vi "ConfigureChannelPhaseStatus.vi"(8 "shared data group exist?":bool, 9 "AssetNodes":T5[](array[typedef]), 10 "AllChannels":T3[](array[typedef]), 11 "ChannelModel":T3) -> (2 "valid":bool, 3 "DataGroup ChannelStatus Out":T1[](array[typedef]))   [LabVIEW 2017, in "McsaTestPanel.lvlib"]
uses:
  <vilib>/addons/InsightCM/Devices/Shared/Mcsa/McsaTestPanel/McsaTestPanel.lvlib
  <vilib>/addons/InsightCM/MessageBus/Base/controls/AssetNode.ctl
  <vilib>/addons/InsightCM/MessageBus/Base/controls/AssetState.ctl
  <vilib>/addons/InsightCM/MessageBus/Base/controls/KeyValuePair.ctl
  <vilib>/addons/InsightCM/MessageBus/Base/controls/OperatingState.ctl
  <vilib>/addons/InsightCM/MessageBus/Base/controls/Trigger.ctl
  <vilib>/addons/InsightCM/MessageBus/Base/controls/Condition.ctl
  <vilib>/addons/InsightCM/MessageBus/Base/controls/Metric.ctl
  <vilib>/addons/InsightCM/MessageBus/Base/controls/TrendAlarmRule.ctl
  <vilib>/addons/InsightCM/MessageBus/Base/controls/TrendAlarmLevel.ctl
  <vilib>/addons/InsightCM/MessageBus/Base/controls/AlarmAction.ctl
  <vilib>/addons/InsightCM/MessageBus/Base/controls/AssetNodeReference.ctl
  <vilib>/addons/InsightCM/MessageBus/Base/controls/R2_Channel.ctl
  <vilib>/addons/InsightCM/Devices/Shared/Mcsa/McsaTestPanel/controls/ChannelStatus.ctl
  <vilib>/addons/InsightCM/Utilities/PropertyHelpers/PropertyHelpers.lvlib
  <vilib>/addons/InsightCM/Utilities/DeviceModelHelpers/DeviceModelHelpers.lvlib
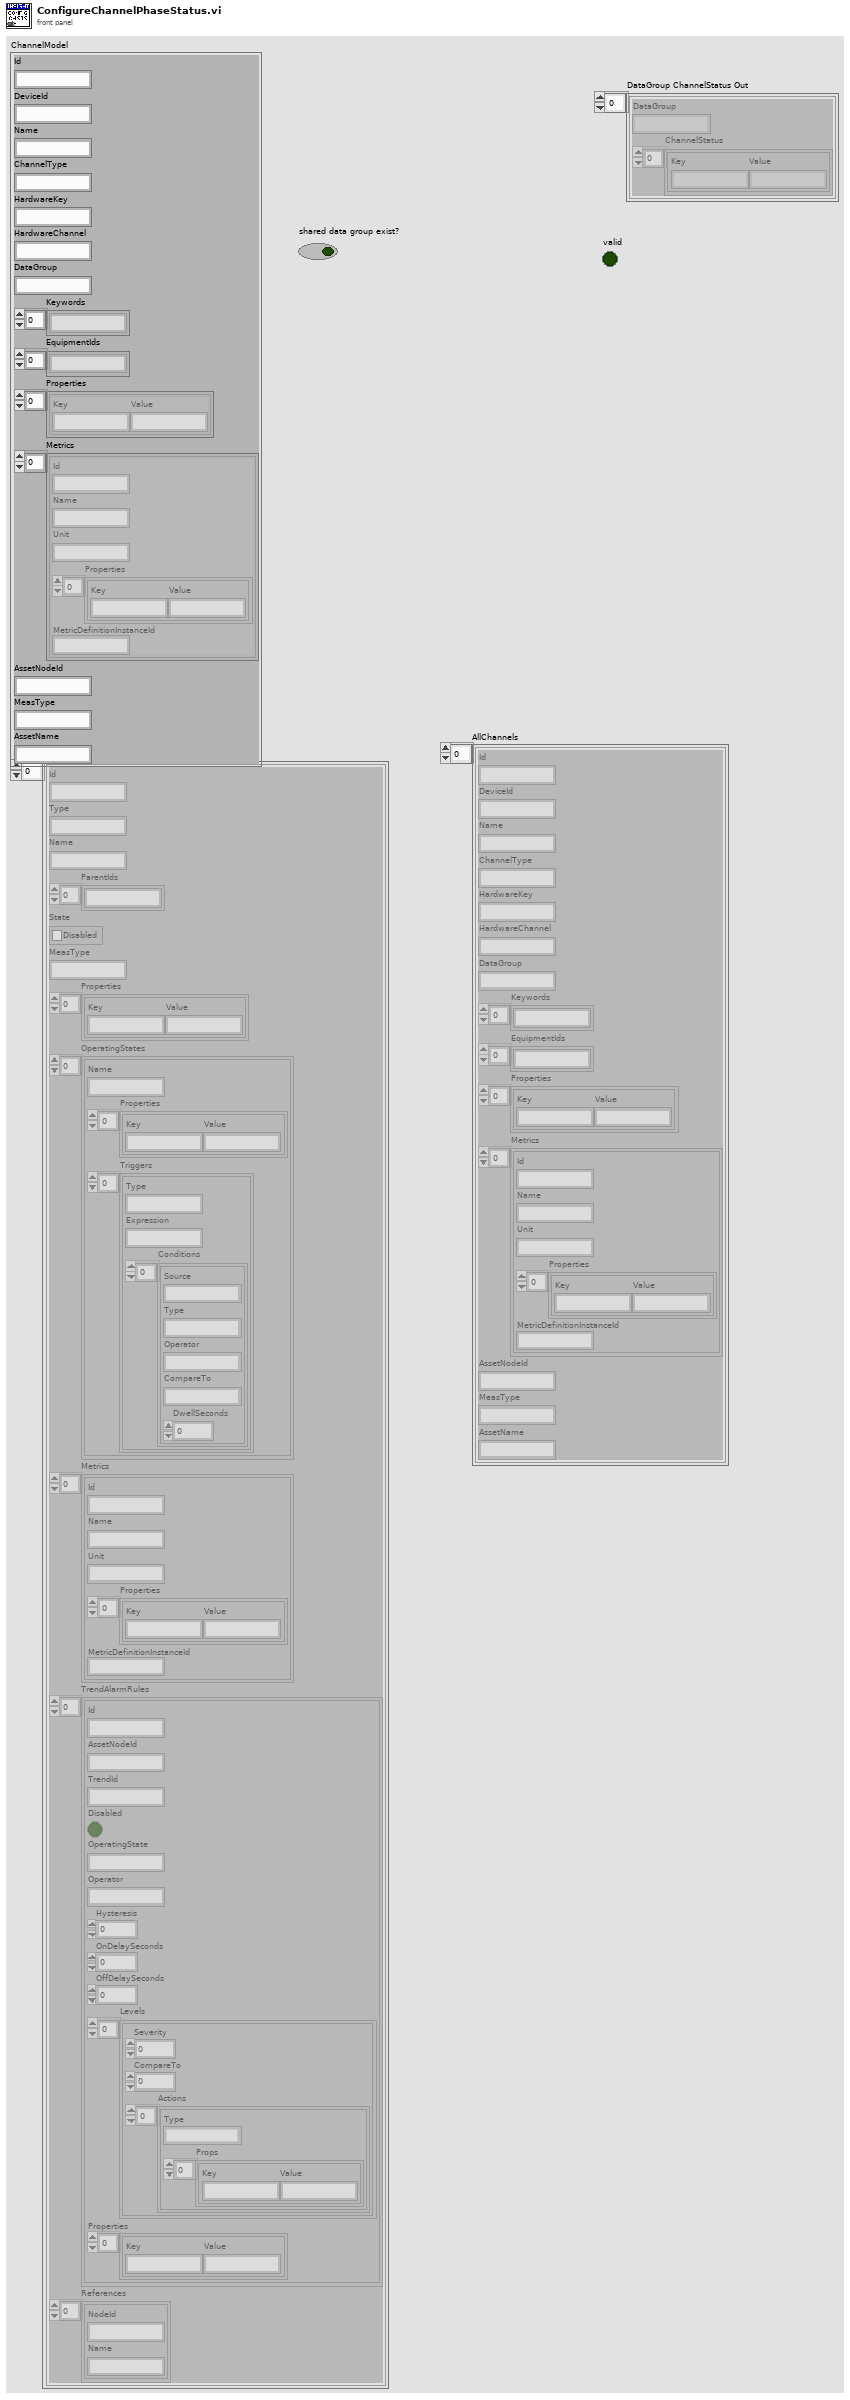
[diagram p1: front panel]
types:
  T1 = typedef "McsaTestPanel.lvlib/ChannelStatus.ctl" = cluster{"DataGroup":string, "ChannelStatus":T2[]}
  T2 = typedef "KeyValuePair.ctl" = cluster{"Key":string, "Value":string}
  T3 = typedef "R2_Channel.ctl" = cluster{"Id":string, "DeviceId":string, "Name":string, "ChannelType":string, "HardwareKey":string, "HardwareChannel":string, "DataGroup":string, "Keywords":string[], "EquipmentIds":string[], "Properties":T2[], "Metrics":T4[], "AssetNodeId":string, "MeasType":string, "AssetName":string}
  T4 = typedef "Metric.ctl" = cluster{"Id":string, "Name":string, "Unit":string, "Properties":T2[], "MetricDefinitionInstanceId":string}
  T5 = typedef "AssetNode.ctl" = cluster{"Id":string, "Type":string, "Name":string, "ParentIds":string[], "State":T6, "MeasType":string, "Properties":T2[], "OperatingStates":T7[], "Metrics":T4[], "TrendAlarmRules":T10[], "References":T13[]}
  T6 = typedef "AssetState.ctl" = cluster{"Disabled":bool}
  T7 = typedef "OperatingState.ctl" = cluster{"Name":string, "Properties":T2[], "Triggers":T8[]}
  T8 = typedef "Trigger.ctl" = cluster{"Type":string, "Expression":string, "Conditions":T9[]}
  T9 = typedef "Condition.ctl" = cluster{"Source":string, "Type":string, "Operator":string, "CompareTo":string, "DwellSeconds":dbl}
  T10 = typedef "TrendAlarmRule.ctl" = cluster{"Id":string, "AssetNodeId":string, "TrendId":string, "Disabled":bool, "OperatingState":string, "Operator":string, "Hysteresis":dbl, "OnDelaySeconds":dbl, "OffDelaySeconds":dbl, "Levels":T11[], "Properties":T2[]}
  T11 = typedef "TrendAlarmLevel.ctl" = cluster{"Severity":i32, "CompareTo":dbl, "Actions":T12[]}
  T12 = typedef "AlarmAction.ctl" = cluster{"Type":string, "Props":T2[]}
  T13 = typedef "AssetNodeReference.ctl" = cluster{"NodeId":string, "Name":string}
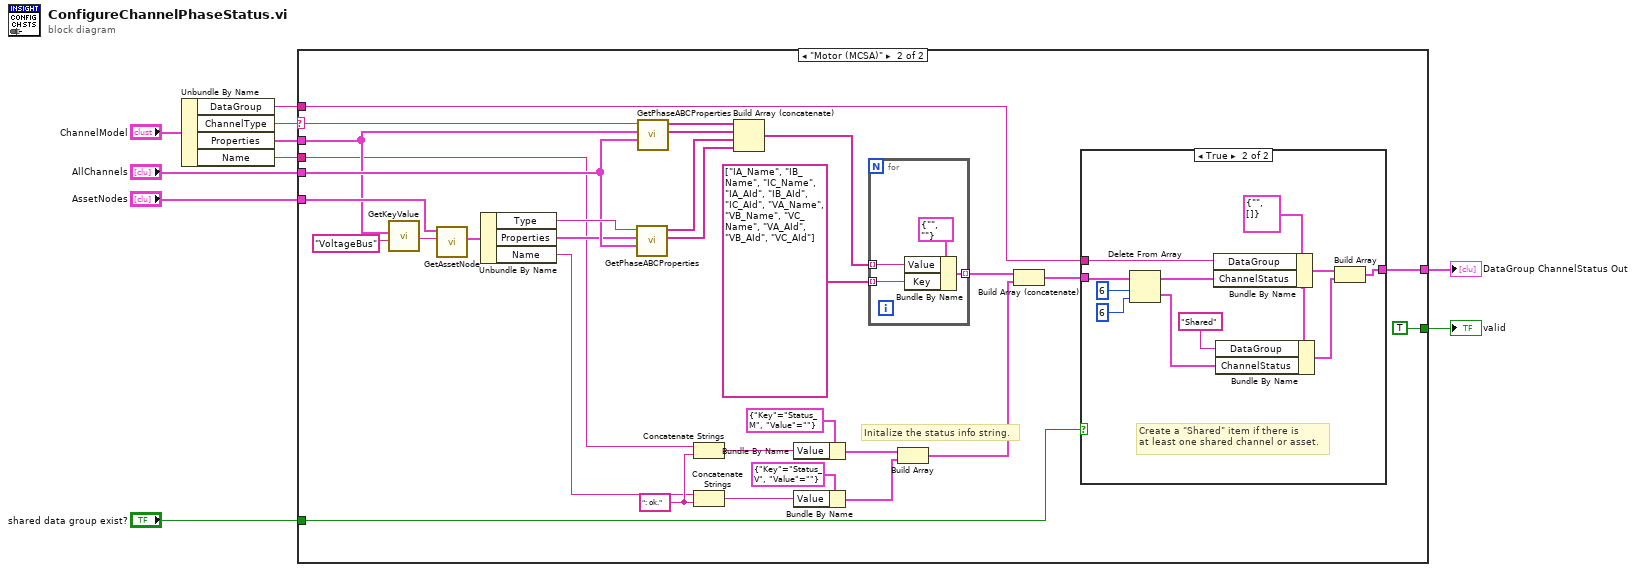
[diagram p0: block diagram]
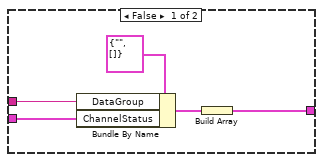
[diagram p3: hidden frame]
diagram:
  n1 = Unbundle By Name("ChannelModel") -> ("DataGroup"=w5:string, "ChannelType"=w6:string, "Properties"=w7:T2[], "Name"=w2:string)
  n2 = case shown="\"Motor (MCSA)\"" w6 {
    selector: w6 -> [_ w41]
    tunnel: w7 -> [_ w35]
    tunnel: "AllChannels" -> [_ w36]
    tunnel: "AssetNodes" -> [_ w39]
    tunnel: w5 -> [_ w13]
    tunnel: [_ w29] -> w3
    tunnel: "shared data group exist?" -> [_ w12]
    tunnel: w2 -> [_ w19]
    tunnel: [_ TRUE ("valid")] -> w1
    frame Default {
    }
    frame "Motor (MCSA)" {
      w20 = ": ok." ("string")
      # "Initalize the status info string."
      n3 = call <vilib>:"GetKeyValue.vi"("key"="VoltageBus", "key value pairs"=w35) -> ("value"=w23:string)  [unwired: 7 in, 2 out]
      n4 = call <vilib>:"GetAssetNode.vi"("node id"=w23, "nodes in"=w39) -> ("AssetNode"=w38:T5)  [unwired: 7 in, 2 out]
      n5 = Unbundle By Name(w38) -> ("Type"=w37:string, "Properties"=w34:T2[], "Name"=w18:string)
      n6 = call <vilib>:"GetPhaseABCProperties.vi"("Channels"=w36, "Channel Properties"=w34, "ChannelType"=w37) -> ("AssetIdABC"=w14:string[], "AssetNameABC"=w15:string[])  [unwired: 6 in, 1 out]
      n7 = call <vilib>:"GetPhaseABCProperties.vi"("Channels"=w36, "Channel Properties"=w35, "ChannelType"=w41) -> ("AssetIdABC"=w16:string[], "AssetNameABC"=w17:string[])  [unwired: 6 in, 1 out]
      n8 = Concatenate Strings(w19, w20) -> (w21:string)
      n9 = Concatenate Strings(w18, w20) -> (w22:string)
      n10 = Build Array (concatenate)(w17, w16, w15, w14) -> (w33:string[])
      n11 = Bundle By Name(cluster=T2 {"Key"="Status_M", "Value"=""}, "Value"=w21) -> (w26:T2)
      n12 = Bundle By Name(cluster=T2 {"Key"="Status_V", "Value"=""}, "Value"=w22) -> (w25:T2)
      n13 = for {
        tunnel: w33 -> [w60] mode=indexing
        tunnel: string[] ["IA_Name", "IB_Name", "IC_Name", "IA_AId", "IB_AId", "IC_AId", "VA_Name", "VB_Name", "VC_Name", "VA_AId", "VB_AId", "VC_AId"] -> [w58] mode=indexing
        tunnel: [w59] -> w31 mode=indexing
        n14 = Bundle By Name(cluster=T2 {"Key"="", "Value"=""}, "Value"=w60, "Key"=w58) -> (w59:T2)
      }
      n15 = Build Array(w26, w25) -> (w24:T2[])
      n16 = Build Array (concatenate)(w31, w24) -> (w30:T2[])
      n17 = case shown="True" w12 {
        tunnel: w13 -> [w44 w57]
        tunnel: w30 -> [w43 w48]
        tunnel: [w42 w55] -> w29
        frame False {
          n18 = Bundle By Name(cluster=T1 {"DataGroup"="", "ChannelStatus"=[]} ("DataGroup ChannelStatus"), "DataGroup"=w44, "ChannelStatus"=w43) -> (w46:T1)
          n19 = Build Array(w46) -> (w42:T1[])
        }
        frame True {
          w54 = T1 {"DataGroup"="", "ChannelStatus"=[]} ("DataGroup ChannelStatus")
          # "Create a \"Shared\" item if there is \nat least one shared channel or asset."
          n20 = Delete From Array(array=w48, length=6 ("index"), index=6 ("length")) -> (deleted portion=w49:T2[], array with subset deleted=w47:T2[])
          n21 = Bundle By Name(cluster=w54, "DataGroup"=w57, "ChannelStatus"=w47) -> (w56:T1)
          n22 = Bundle By Name(cluster=w54, "DataGroup"="Shared", "ChannelStatus"=w49) -> (w53:T1)
          n23 = Build Array(w56, w53) -> (w55:T1[])
        }
      }
    }
  }
  "DataGroup ChannelStatus Out" <- w3
  "valid" <- w1
